vi "TSE_Variables.vi"() -> ()   [LabVIEW 2014]
uses:
  CustomControls/User_Selection.ctl
  CustomControls/TSE_Status.ctl
  CustomControls/Program_States.ctl
panel:
  in  "Uygulanan_Deger":dbl[](array[numeric])
  in  "TSE Status":T1={"Return Code"=0, "Message"="", "error in (no error)"={"status"=FALSE, "code"=0, "source"=""}, "Program State"=enum."Ön Yükleme Tamam", "Test A. Suresi"=0}
  in  "TS_Executing":bool
  in  "StopTSE":bool
  in  "Ref_Seri_No":string
  in  "Operator":string
  in  "OlcumNo":u16
  in  "OlcumFonksiyonu":T3=enum."Frekans"
  in  "GPIB_Interface_No":string
  in  "GKC_Uretici":string
  in  "ExecuteTest":bool
  in  "Cihazin_Sahibi":string
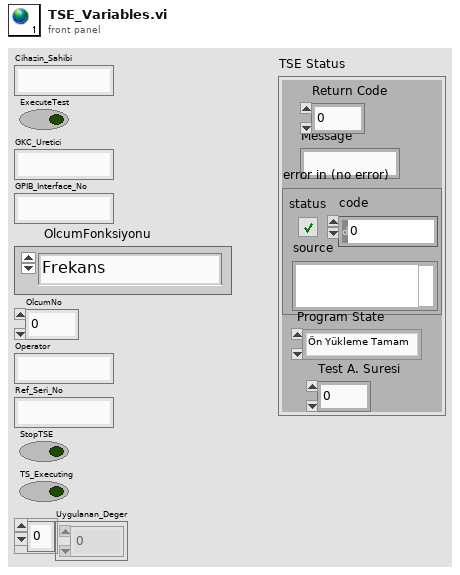
[diagram p1: front panel]
types:
  T1 = typedef "TSE_Status.ctl" = cluster{"Return Code":i32, "Message":string, "error in (no error)":errorcluster, "Program State":T2, "Test A. Suresi":u32}
  T2 = typedef "Program_States.ctl" = enum16{"Ön Yükleme", "TSE Baslat", "Kalibratöre Baglan", "Kalibratörü Baslat", "Ön Yükleme Tamam", "Frekans Testi", "Gerilim Testi", "Akim Testi", "Aktif Guc Testi", "Reaktif Guc Testi", "AC Akim Harmonik Testi", "AC Gerilim Harmonik Testi", "Flicker Testi", "Rapor Cikarma", "Yeniden Başlat", "Bekleme", "Durdur"}
  T3 = typedef "User_Selection.ctl" = enum16{"Tüm Fonksiyonlar", "Frekans", "AC Gerilim", "AC Akım", "Aktif Güç", "Reaktif Güç", "Harmonik Akım", "Harmonik Gerilim", "Flicker", "Sertifika Oluştur"}
diagram:
